vi "IMAQDevice.add_Services.vi"(0 "i ref in":refnum<vi>, 5 "error in (no error)":errorcluster) -> (14 "i ref out":refnum<vi>, 19 "error out":errorcluster)   [LabVIEW 2014, in "IMAQDevice.lvlib"]
doc: "ThisVI adds the DIM services to the server. The number of services depends on the maximum size per service (fixed to 250kByte) and the size of the image.\n\nLicense Agreement for this software:\n\nCopyright (C)\nGesellschaft für Schwerionenforschung, GSI\nPlanckstr. 1\n64291 Darmstadt\nGermany\n\nContact: D.Beck@gsi.de \n\nThis program is free software; you can redistribute it and/or modify it under the terms of the \nGNU General Public License as published by the Free Software Foundation; either version 2 of \nthe license, or (at your option) any later version.\n\nThis program is distributed in the hope that it will be useful, but WITHOUT ANY WARRANTY; \nwithout even the implied warranty of MERCHANTABILITY or FITNESS FOR A PARTICULAR PURPOSE. See the GNU General License for more details (http://www.gnu.org).\n\nGesellschaft für Schwerionenforschung, GSI\nPlanckstr. 1, 64291 Darmstadt, Germany\nFor all questions and ideas contact: M.Richter@gsi.de, H.Brand@gsi.de or D.Beck@gsi.de.\nLast update: 16-JUN-2004"
uses:
  IMAQDevice.lvlib
  CSlibraries-extern/DimLVEvent/LVDimInterface/LVDimInterface.lvlib
  CSCore/CSSystem/CSSystemLib/CSSystemLib.lvlib
  CSlibraries/UtilityLib/UtilityLib.lvlib
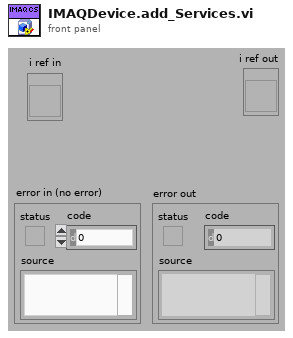
[diagram p1: front panel]
types:
  T1 = typedef "IMAQDevice.lvlib/IMAQDevice.i attribute.ctl" = cluster{"HGF_IMAQ.lvlib:HGF_IMAQDevice.lvclass":refnum<class "HGF_IMAQDevice.lvclass">, "Image":T2, "TimeStampID":i32, "Image IDs":i32[], "NumberOfImagesID":i32, "JPEG?":bool, "JPEGID":i32, "JPEG_ImageID":i32, "TriggerModeID":i32, "OffsetFromLeft":i32, "OffsetFromTop":i32, "HorizontalPixelPerMm":dbl, "VerticalPixelPerMm":dbl, "Grid":cluster{"1":cluster{i32, i32}, "2":cluster{i32, i32}, "3":cluster{i32, i32}, "4":cluster{i32, i32}}, "GridR":cluster{"1":cluster{dbl, dbl}, "2":cluster{dbl, dbl}, "3":cluster{dbl, dbl}, "4":cluster{dbl, dbl}}, "CameraTypeID":i32, "CameraInfos":cluster{"Camera Name-Array":string[], "own Camera Type":string}, "TakeMeasurement?":bool, "TriggerArmedID":i32, "Mirroring":i16, "Rotation":dbl}
  T2 = typedef "IMAQ Image.ctl" = refnum<image>
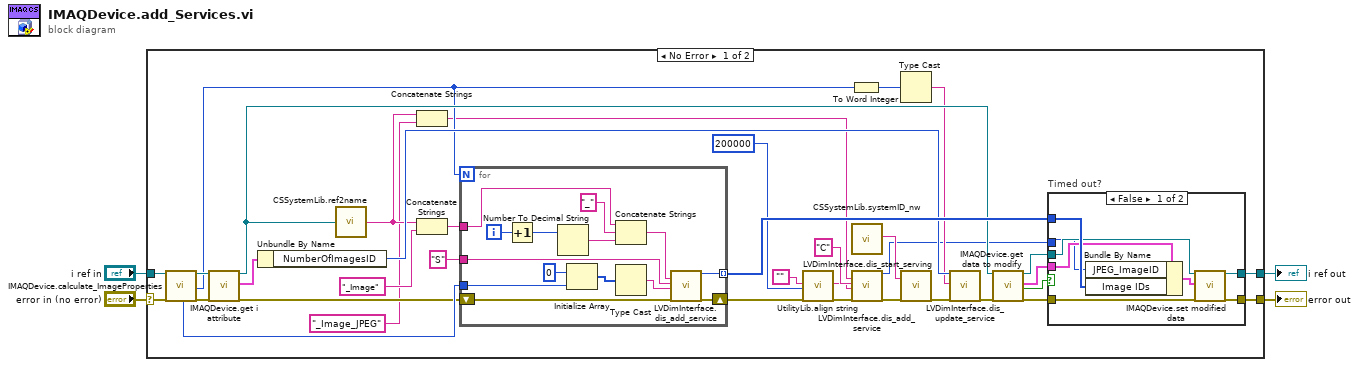
[diagram p0: block diagram]
diagram:
  n1 = case shown="No Error" "error in (no error)" {
    selector: "error in (no error)" -> [w32 w66]
    tunnel: "i ref in" -> [w33 w65]
    tunnel: [w35 w66] -> w2
    tunnel: [w36 w65] -> w1
    frame No Error {
      n2 = call "IMAQDevice.calculate_ImageProperties.vi"("i ref in"=w33, "error in (no error)"=w32) -> ("length per DIM service / 16 Bit"=w27:i32, "i ref out"=w23:refnum<vi>, "number of DIM services"=w17:u8, "error out"=w24:errorcluster)  [unwired: 8 in, 6 out]
      n3 = call "IMAQDevice.get i attribute.vi"("i ref in"=w23, "error in (no error)"=w24) -> ("i ref out"=w22:refnum<vi>, "i attribute"=w20:T1, "error out"=w21:errorcluster)  [unwired: 15 in]
      n4 = Unbundle By Name(w20) -> ("NumberOfImagesID"=w19:i32)
      n5 = call "CSSystemLib.ref2name.vi"("obj refnum"=w22) -> ("name"=w13:string)
      n6 = Concatenate Strings(w13, "_Image_JPEG" ("string")) -> (w11:string)
      n7 = Concatenate Strings(w13, "_Image" ("string")) -> (w40:string)
      n8 = for {
        N: w17 -> [_]
        tunnel: [w64] -> w37 mode=indexing
        tunnel: w40 -> [w59]
        tunnel: "S" ("typeDescriptor") -> [w63]
        shift-right: [w62] -> w8
        shift-left: w21 -> [w61]
        tunnel: w27 -> [w53]
        i -> [w56]
        n9 = Increment(x=w56) -> (x+1=w52:i32)
        n10 = Number To Decimal String(number=w52) -> (decimal integer string=w57:string)  [unwired: 1 in]
        n11 = Initialize Array(u16 0 ("x"), w53) -> (w55:u16[])
        n12 = Concatenate Strings(w59, "_", w57) -> (w60:string)
        n13 = Type Cast(x=w55) -> (*(type *) &x=w54:string)  [unwired: 1 in]
        n14 = call "LVDimInterface.dis_add_service.vi"("serviceName"=w60, "typeDescriptor"=w63, "data"=w54, "error in (no error)"=w61) -> ("my_serviceID"=w64:i32, "error out"=w62:errorcluster)  [unwired: 14 in]
      }
      n15 = call "UtilityLib.align string.vi"("stringIn"="", "stringLength (80)"=200000, "error in (no error)"=w8) -> ("stringOut"=w7:string, "error out"=w9:errorcluster)  [unwired: 15 in]
      n16 = To Word Integer(number=w17) -> (16bit integer=w16:i16)
      n17 = call "CSSystemLib.systemID_nw.vi"() -> ("systemID out"=w34:string)  [unwired: 18 in, 1 out]
      n18 = call "LVDimInterface.dis_add_service.vi"("serviceName"=w11, "typeDescriptor"="C", "data"=w7, "error in (no error)"=w9) -> ("my_serviceID"=w15:i32, "error out"=w14:errorcluster)  [unwired: 14 in]
      n19 = Type Cast(x=w16) -> (*(type *) &x=w18:string)  [unwired: 1 in]
      n20 = call "LVDimInterface.dis_start_serving.vi"("serverName"=w34, "error in (no error)"=w14) -> ("error out"=w26:errorcluster)  [unwired: 16 in, 1 out]
      n21 = call "LVDimInterface.dis_update_service.vi"("my_serviceID"=w19, "data"=w18, "error in (no error)"=w26) -> ("error out"=w25:errorcluster)  [unwired: 14 in, 2 out]
      n22 = call "IMAQDevice.get data to modify.vi"("i ref in"=w22, "error in (no error)"=w25) -> ("i ref out"=w30:refnum<vi>, "i attribute"=w29:T1, "timed out"=w28:bool, "error out"=w31:errorcluster)  [unwired: 14 in]
      n23 = case "Timed out?" shown="False" w28 {
        tunnel: w37 -> [w48 _]
        tunnel: [w47 w50] -> w36
        tunnel: [w46 w49] -> w35
        tunnel: w31 -> [w45 w49]
        tunnel: w30 -> [w44 w50]
        tunnel: w29 -> [w43 _]
        tunnel: w15 -> [w41 _]
        frame False {
          n24 = Bundle By Name(cluster=w43, "JPEG_ImageID"=w41, "Image IDs"=w48) -> (w42:T1)
          n25 = call "IMAQDevice.set modified data.vi"("i ref in"=w44, "i attribute"=w42, "error in (no error)"=w45) -> ("i ref out"=w47:refnum<vi>, "error out"=w46:errorcluster)  [unwired: 15 in]
        }
        frame True {
        }
      }
    }
    frame Error {
    }
  }
  "i ref out" <- w1
  "error out" <- w2
